vi "EnqueueWithParameter.vi"(8 "Parameter":variant, 9 "Command":T1, 11 "Command Q":refnum<queue>) -> (3 "Command Q":refnum<queue>)   [LabVIEW 2014]
doc: "Enqueues job for the consumer's state machine.\n\nAny parameter can be passed via the variant. To avoid conflicts, all front panel items should be passed from the producer to the consumer via this variant, and not, for example, through local variables."
uses:
  Controls/ExperimentControlEnum.ctl
  Controls/ExperimentControlCluster.ctl
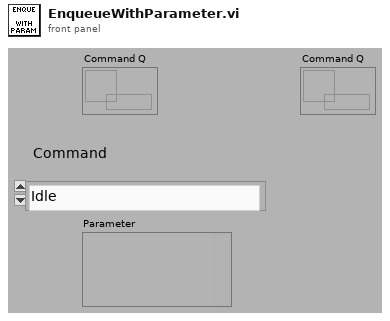
[diagram p1: front panel]
types:
  T1 = typedef "ExperimentControlEnum.ctl" = enum16{"Idle", "FIRE: Read Panel Settings", "FIRE: Generate Tasks", "FIRE: Set DAQ Triggers", "FIRE: Trigger", "FIRE: Wait for Task Completion", "FIRE: Read out Digitizers", "FIRE: Write to MDS+", "Save shot quality", "Discard shot data", "Clear Tasks", "Stop VI", "DIO Change", "Update Tree", "Load Shot Settings", "Restore Default Settings", "Store Scope Data", "Store Camera Data", "Tach Change"}
  T2 = typedef "ExperimentControlCluster.ctl" = cluster{"Experiment Control":T1, "Variant":variant}
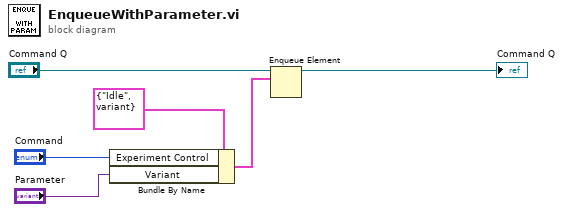
[diagram p0: block diagram]
diagram:
  n1 = Bundle By Name(cluster=T2 {"Experiment Control"=enum."Idle", "Variant"=variant} ("element"), "Experiment Control"="Command", "Variant"="Parameter") -> (w6:T2)
  n2 = Enqueue Element(queue="Command Q", element=w6) -> (queue out=→"Command Q":refnum<queue>)  [unwired: 1 in, 3 out]
